vi "read.vi"(8 "error in (no error)":errorcluster, 10 "timeout (ms)":i32=500, 11 "CEG4500 in":refnum<class "CEG4500.lvclass">) -> (0 "error out":errorcluster, 2 "Return String":string, 3 "CEG4500 out":refnum<class "CEG4500.lvclass">)   [LabVIEW 2013, in "CEG4500.lvclass"]
uses:
  CEG4500.lvclass
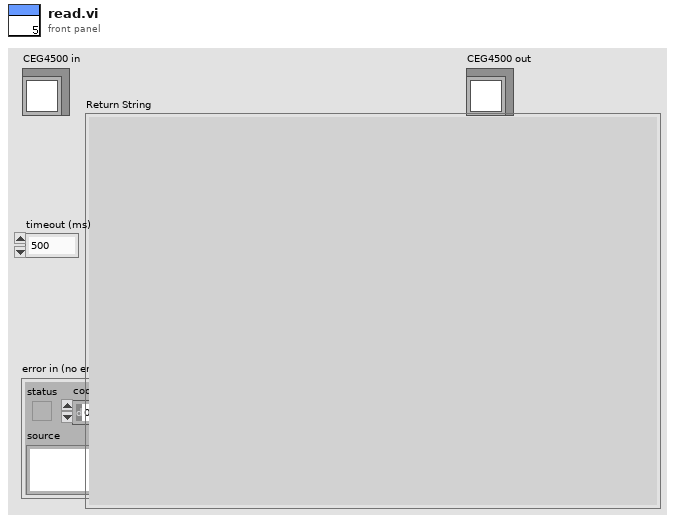
[diagram p1: front panel]
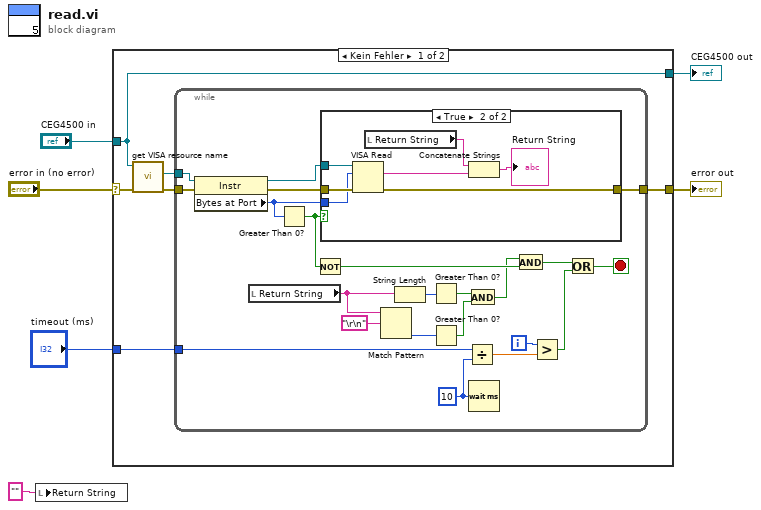
[diagram p0: block diagram]
diagram:
  n1 = local write "Return String"("" ("Return String")) -> ()
  n2 = case shown="Kein Fehler" "error in (no error)" {
    selector: "error in (no error)" -> [w10 w44]
    tunnel: [w12 w44] -> w4
    tunnel: [w8 w43] -> w2
    tunnel: "CEG4500 in" -> [w8 w43]
    tunnel: "timeout (ms)" -> [w11 _]
    frame No Error {
      n3 = call-dynamic "get VISA resource name.vi"("error in (no error)"=w10, "DeviceInterface (Eingang)"=w8) -> ("error out"=w9:errorcluster, "VISA resource name"=w7:refnum<visa-resource-name>)  [unwired: 7 in, 1 out]
      n4 = while {
        tunnel: [w34] -> w12
        tunnel: w11 -> [w30]
        tunnel: w9 -> [w20]
        tunnel: w7 -> [w19]
        i -> [w27]
        stop <- w25 stop-if-true
        w29 = u32 10 ("milliseconds to wait")
        n5 = property class="Instr"(reference=w19, error in=w20) -> (reference out=w32:refnum<visa-resource-name>, error out=w33:errorcluster, "Bytes at Port"=w31:u32)
        n6 = local read "Return String"() -> (w18:string)
        n7 = Greater Than 0?(x=w31) -> (x > 0?=w23:bool)
        n8 = Not(x=w23) -> (.not. x?=w22:bool)
        n9 = case shown="True" w23 {
          tunnel: [w35 w42] -> w34
          tunnel: w33 -> [w35 w39]
          tunnel: w31 -> [_ w38]
          tunnel: w32 -> [_ w37]
          frame False {
          }
          frame True {
            n10 = VISA Read(VISA resource name=w37, byte count=w38, error in (no error)=w39) -> (read buffer=w40:string, error out=w42:errorcluster)  [unwired: 2 out]
            n11 = local read "Return String"() -> (w41:string)
            n12 = Concatenate Strings(w41, w40) -> (→"Return String":string)
          }
        }
        n13 = Match Pattern(string=w18, regular expression="\r\n") -> (offset past match=w16:i32)  [unwired: 1 in, 3 out]
        n14 = String Length(string=w18) -> (length=w24:i32)
        n15 = Greater Than 0?(x=w24) -> (x > 0?=w14:bool)
        n16 = Greater Than 0?(x=w16) -> (x > 0?=w15:bool)
        n17 = Divide(x=w30, y=w29) -> (x/y=w28:dbl)
        n18 = And(x=w14, y=w15) -> (x .and. y?=w13:bool)
        n19 = Wait (ms)(milliseconds to wait=w29) -> ()  [unwired: 1 out]
        n20 = And(x=w13, y=w22) -> (x .and. y?=w21:bool)
        n21 = Greater?(x=w27, y=w28) -> (0:w26:bool)
        n22 = Or(x=w21, y=w26) -> (x .or. y?=w25:bool)
      }
    }
    frame Error {
    }
  }
  "error out" <- w4
  "CEG4500 out" <- w2
